vi "Process.vi"(8 "error in (no error)":errorcluster, 11 "Coverage Analyzer In":refnum<class "Coverage Analyzer Process.lvclass">) -> (0 "error out":errorcluster, 3 "Coverage Analyzer Out":refnum<class "Coverage Analyzer Process.lvclass">)   [LabVIEW 2020, in "Coverage Analyzer Process.lvclass"]
uses:
  Coverage Analyzer Process.lvclass
  C:/git/astemes-lunit/source/User Interface/Process/Process.lvclass
  User Interface/Process/Process.lvclass/Process.ctl
  Coverage Analyzer Process.lvclass/Coverage Analyzer Process.ctl
  <vilib>/Utility/error.llb/Error Cluster From Error Code.vi
  <vilib>/ErrorRing/Error Ring.xnode
  User Interface/Process/Process.lvclass
  Coverage Analyzer/Coverage Analyzer.lvclass
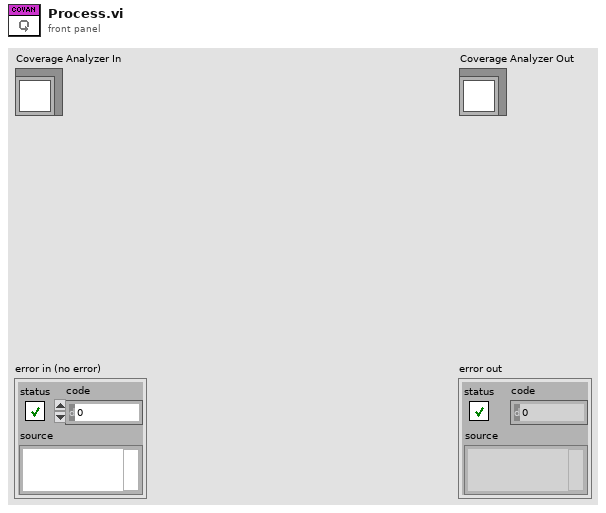
[diagram p1: front panel]
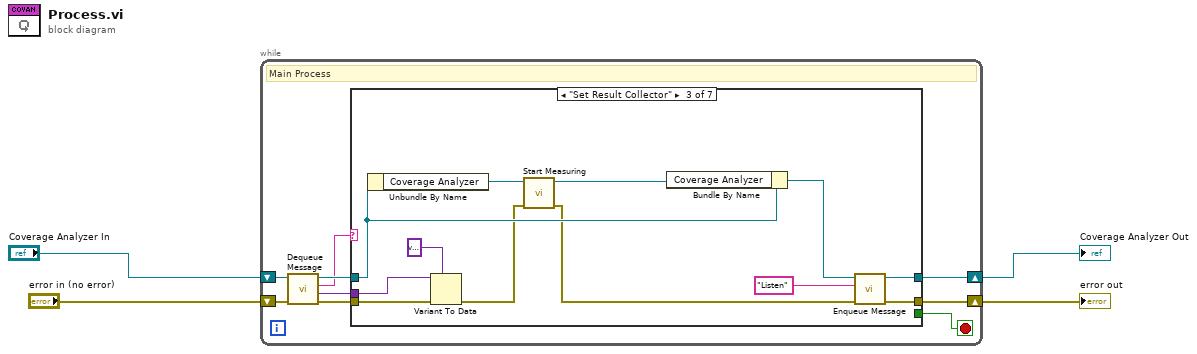
[diagram p0: block diagram]
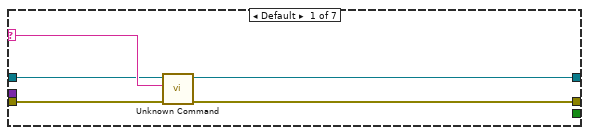
[diagram p2: hidden frame]
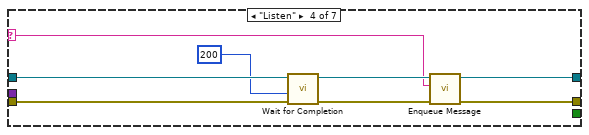
[diagram p4: hidden frame]
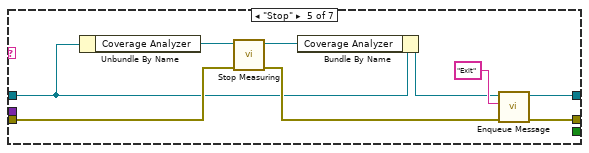
[diagram p5: hidden frame]
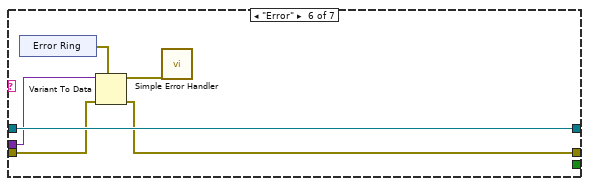
[diagram p6: hidden frame]
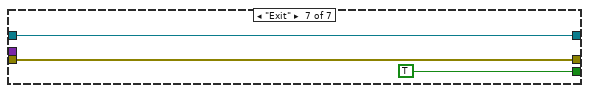
[diagram p7: hidden frame]
diagram:
  n1 = while {
    shift-right: [w8] -> w4
    shift-left: "error in (no error)" -> [w12]
    shift-right: [w10] -> w3
    shift-left: "Coverage Analyzer In" -> [w13]
    stop <- w5 stop-if-true
    # "Main Process"
    n2 = call "Dequeue Message.vi"("error in (no error)"=w12, "Process In"=w13) -> ("error out"=w11:errorcluster, "Message Data"=w6:variant, "Message"=w7:string, "Process Out"=w9:refnum<class "Coverage Analyzer Process.lvclass">)  [unwired: 6 in]
    n3 = case shown="\"Set Result Collector\"" w7 {
      selector: w7 -> [w18 _ _ w34 _ _ _]
      tunnel: [w15 w19 w25 w37 w48 w51 w57] -> w8
      tunnel: w11 -> [w14 w19 w32 w39 w45 w54 w57]
      tunnel: [w17 w20 w28 w35 w47 w55 w58] -> w10
      tunnel: w9 -> [w16 w20 w27 w40 w43 w55 w58]
      tunnel: w6 -> [_ _ w31 _ _ w53 _]
      tunnel: [_ _ _ _ _ _ TRUE] -> w5
      frame Default {
        n4 = call "Unknown Command.vi"("error in (no error)"=w14, "String"=w18, "Process In"=w16) -> ("error out"=w15:errorcluster, "Process Out"=w17:refnum<class "Coverage Analyzer Process.lvclass">)  [unwired: 7 in]
      }
      frame "Init" {
      }
      frame "Set Result Collector" {
        n5 = Unbundle By Name(w27) -> ("Coverage Analyzer"=w26:refnum<class "Coverage Analyzer.lvclass">)
        n6 = Variant To Data(error in=w32, type=variant, Variant=w31) -> (error out=w23:errorcluster)  [unwired: 1 out]
        n7 = call "Start Measuring.vi"("error in (no error)"=w23, "Coverage Analyzer in"=w26) -> ("error out"=w22:errorcluster, "Coverage Analyzer out"=w24:refnum<class "Coverage Analyzer.lvclass">)  [unwired: 8 in]
        n8 = Bundle By Name(cluster=w27, "Coverage Analyzer"=w24) -> (w30:refnum<class "Coverage Analyzer Process.lvclass">)
        n9 = call "Enqueue Message.vi"("error in (no error)"=w22, "Message"="Listen", "Process In"=w30) -> ("error out"=w25:errorcluster, "Process Out"=w28:refnum<class "Coverage Analyzer Process.lvclass">)  [unwired: 7 in]
      }
      frame "Listen" {
        n10 = call "Wait for Completion.vi"("error in (no error)"=w39, "Timeout"=200, "Coverage Analyzer Process in"=w40) -> ("error out"=w38:errorcluster, "Coverage Analyzer Process out"=w36:refnum<class "Coverage Analyzer Process.lvclass">)  [unwired: 7 in]
        n11 = call "Enqueue Message.vi"("error in (no error)"=w38, "Message"=w34, "Process In"=w36) -> ("error out"=w37:errorcluster, "Process Out"=w35:refnum<class "Coverage Analyzer Process.lvclass">)  [unwired: 7 in]
      }
      frame "Stop" {
        n12 = Unbundle By Name(w43) -> ("Coverage Analyzer"=w42:refnum<class "Coverage Analyzer.lvclass">)
        n13 = call "Stop Measuring.vi"("error in (no error)"=w45, "Coverage Analyzer in"=w42) -> ("error out"=w46:errorcluster, "Coverage Analyzer out"=w41:refnum<class "Coverage Analyzer.lvclass">)  [unwired: 8 in]
        n14 = Bundle By Name(cluster=w43, "Coverage Analyzer"=w41) -> (w44:refnum<class "Coverage Analyzer Process.lvclass">)
        n15 = call "Enqueue Message.vi"("error in (no error)"=w46, "Message"="Exit", "Process In"=w44) -> ("error out"=w48:errorcluster, "Process Out"=w47:refnum<class "Coverage Analyzer Process.lvclass">)  [unwired: 7 in]
      }
      frame "Error" {
        n16 = xnode "Error Ring"() -> ("error out"=w52:errorcluster)
        n17 = Variant To Data(error in=w54, type=w52, Variant=w53) -> (data=w50:errorcluster, error out=w51:errorcluster)
        n18 = call <vilib>:"Simple Error Handler.vi"("error in (no error)"=w50) -> ()  [unwired: 4 in, 5 out]
      }
      frame "Exit" {
      }
    }
  }
  "error out" <- w4
  "Coverage Analyzer Out" <- w3
